vi "Result To Error.vi"(8 "error in (no error)":errorcluster, 11 "Result Code":i32) -> (0 "error out":errorcluster)   [LabVIEW 2020, in "G-Audio.lvlib"]
doc: "Converts the result codes found in g_audio.h to a custom LabVIEW error code. The custom error code range begins at 559240."
uses:
  G-Audio.lvlib
  <vilib>/Utility/error.llb/Error Cluster From Error Code.vi
  <vilib>/ErrorRing/Error Ring.xnode
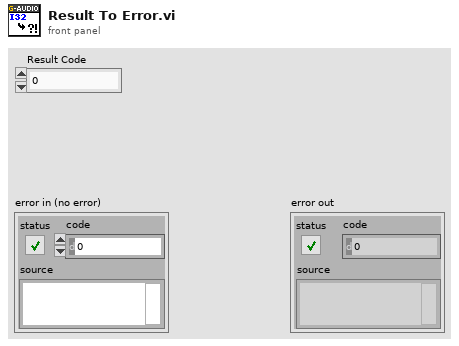
[diagram p1: front panel]
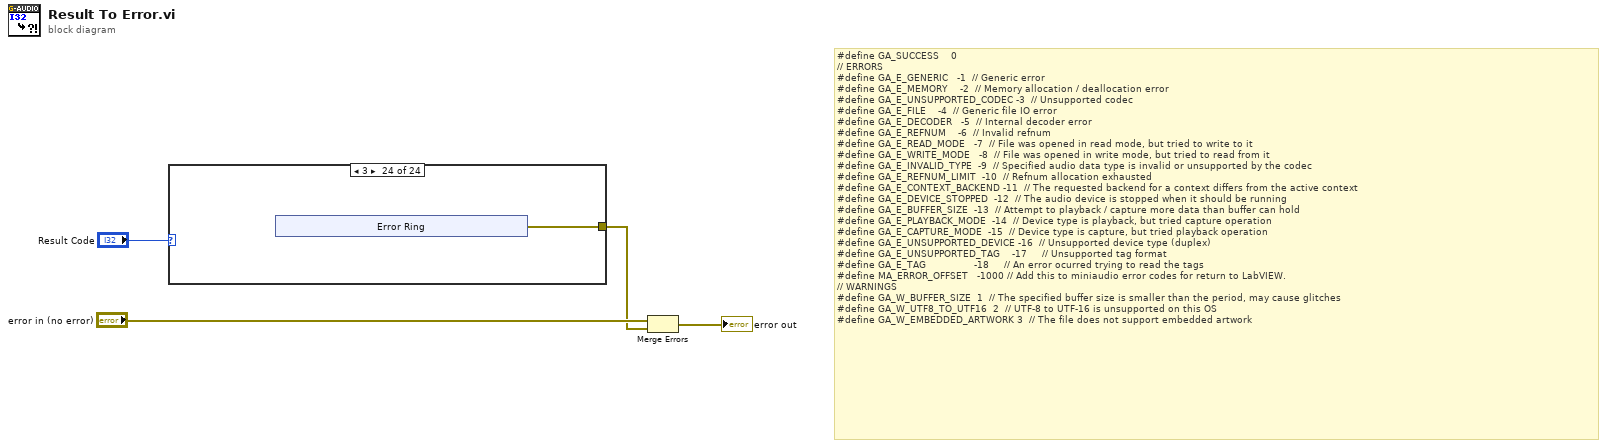
[diagram p0: block diagram]
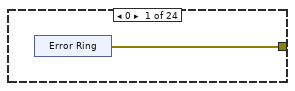
[diagram p2: hidden frame]
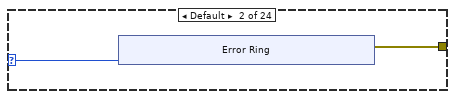
[diagram p3: hidden frame]
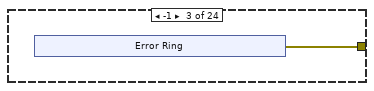
[diagram p4: hidden frame]
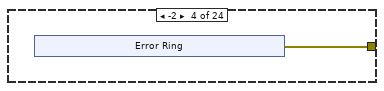
[diagram p5: hidden frame]
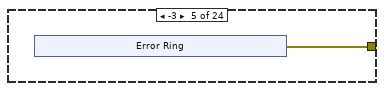
[diagram p6: hidden frame]
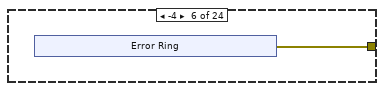
[diagram p7: hidden frame]
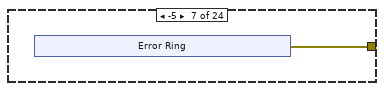
[diagram p8: hidden frame]
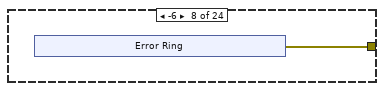
[diagram p9: hidden frame]
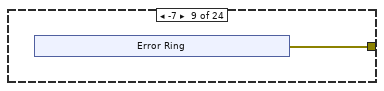
[diagram p10: hidden frame]
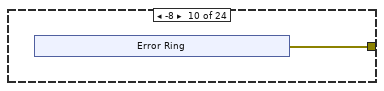
[diagram p11: hidden frame]
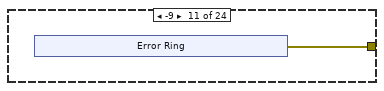
[diagram p12: hidden frame]
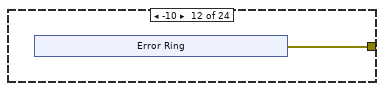
[diagram p13: hidden frame]
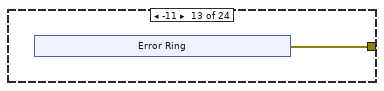
[diagram p14: hidden frame]
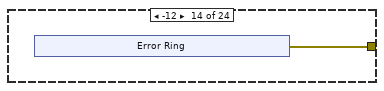
[diagram p15: hidden frame]
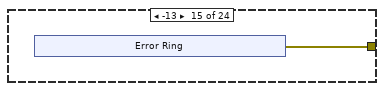
[diagram p16: hidden frame]
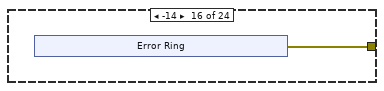
[diagram p17: hidden frame]
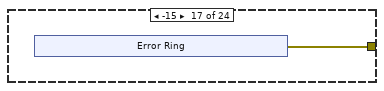
[diagram p18: hidden frame]
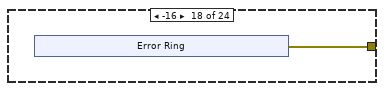
[diagram p19: hidden frame]
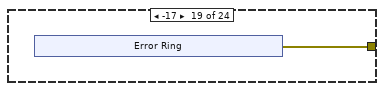
[diagram p20: hidden frame]
diagram:
  # "#define GA_SUCCESS\t\t\t\t0\n// ERRORS\n#define GA_E_GENERIC\t\t\t-1\t\t// Generic error\n#define GA_E_MEMORY\t\t\t\t-2\t\t// Memory allocation / deallocation error\n#define GA_E_UNSUPPORTED_CODEC\t-3\t\t// Unsupported codec\n#define GA_E_FILE\t\t\t\t-4\t\t// Generic file IO error\n#define GA_E_DECODER\t\t\t-5\t\t// Internal decoder error\n#define GA_E_REFNUM\t\t\t\t-6\t\t// Invalid refnum\n#define GA_E_READ_MODE\t\t\t-7\t\t// File was opened in read mode, but tried to write to it\n#define GA_E_WRITE_MODE\t\t\t-8\t\t// File was opened in write mode, but tried to read from it\n#define GA_E_INVALID_TYPE\t\t-9\t\t// Specified audio data type is invalid or unsupported by the codec\n#define GA_E_REFNUM_LIMIT\t\t-10\t\t// Refnum allocation exhausted\n#define GA_E_CONTEXT_BACKEND\t-11\t\t// The requested backend for a context differs from the active context\n#define GA_E_DEVICE_STOPPED\t\t-12\t\t// The audio device is stopped when it should be running\n#define GA_E_BUFFER_SIZE\t\t-13\t\t// Attempt to playback / capture more data than buffer can hold\n#define GA_E_PLAYBACK_MODE\t\t-14\t\t// Device type is playback, but tried capture operation\n#define GA_E_CAPTURE_MODE\t\t-15\t\t// Device type is capture, but tried playback operation\n#define GA_E_UNSUPPORTED_DEVICE\t-16\t\t// Unsupported device type (duplex)\n#define GA_E_UNSUPPORTED_TAG    -17     // Unsupported tag format\n#define GA_E_TAG                -18     // An error ocurred trying to read the tags\n#define MA_ERROR_OFFSET\t\t\t-1000\t// Add this to miniaudio error codes for return to LabVIEW.\n// WARNINGS\n#define GA_W_BUFFER_SIZE\t\t1\t\t// The specified buffer size is smaller than the period, may cause glitches\n#define GA_W_UTF8_TO_UTF16\t\t2\t\t// UTF-8 to UTF-16 is unsupported on this OS\n#define GA_W_EMBEDDED_ARTWORK\t3\t\t// The file does not support embedded artwork"
  n1 = case shown="3" "Result Code" {
    selector: "Result Code" -> [_ w7 _ _ _ _ _ _ _ _ _ _ _ _ _ _ _ _ _ _ w126 _ _ _]
    tunnel: [w5 w8 w16 w22 w28 w34 w40 w46 w52 w58 w64 w70 w76 w82 w88 w94 w100 w106 w112 w118 w127 w135 w141 w147] -> w1
    frame 0 {
      n2 = xnode "Error Ring"() -> ("error out"=w5:errorcluster)
    }
    frame Default {
      n3 = xnode "Error Ring"("parameter 0"=w7) -> ("error out"=w8:errorcluster)
    }
    frame -1 {
      n4 = xnode "Error Ring"() -> ("error out"=w16:errorcluster)
    }
    frame -2 {
      n5 = xnode "Error Ring"() -> ("error out"=w22:errorcluster)
    }
    frame -3 {
      n6 = xnode "Error Ring"() -> ("error out"=w28:errorcluster)
    }
    frame -4 {
      n7 = xnode "Error Ring"() -> ("error out"=w34:errorcluster)
    }
    frame -5 {
      n8 = xnode "Error Ring"() -> ("error out"=w40:errorcluster)
    }
    frame -6 {
      n9 = xnode "Error Ring"() -> ("error out"=w46:errorcluster)
    }
    frame -7 {
      n10 = xnode "Error Ring"() -> ("error out"=w52:errorcluster)
    }
    frame -8 {
      n11 = xnode "Error Ring"() -> ("error out"=w58:errorcluster)
    }
    frame -9 {
      n12 = xnode "Error Ring"() -> ("error out"=w64:errorcluster)
    }
    frame -10 {
      n13 = xnode "Error Ring"() -> ("error out"=w70:errorcluster)
    }
    frame -11 {
      n14 = xnode "Error Ring"() -> ("error out"=w76:errorcluster)
    }
    frame -12 {
      n15 = xnode "Error Ring"() -> ("error out"=w82:errorcluster)
    }
    frame -13 {
      n16 = xnode "Error Ring"() -> ("error out"=w88:errorcluster)
    }
    frame -14 {
      n17 = xnode "Error Ring"() -> ("error out"=w94:errorcluster)
    }
    frame -15 {
      n18 = xnode "Error Ring"() -> ("error out"=w100:errorcluster)
    }
    frame -16 {
      n19 = xnode "Error Ring"() -> ("error out"=w106:errorcluster)
    }
    frame -17 {
      n20 = xnode "Error Ring"() -> ("error out"=w112:errorcluster)
    }
    frame -18 {
      n21 = xnode "Error Ring"() -> ("error out"=w118:errorcluster)
    }
    frame ..-1000 {
      n22 = Add(x=w126, y=1000) -> (x+y=w125:i32)
      n23 = xnode "Error Ring"("parameter 0"=w125) -> ("error out"=w127:errorcluster)
    }
    frame 1 {
      n24 = xnode "Error Ring"() -> ("error out"=w135:errorcluster)
    }
    frame 2 {
      n25 = xnode "Error Ring"() -> ("error out"=w141:errorcluster)
    }
    frame 3 {
      n26 = xnode "Error Ring"() -> ("error out"=w147:errorcluster)
    }
  }
  n27 = Merge Errors("error in (no error)", w1) -> (→"error out":errorcluster)
